vi "Linearity.vi"() -> ()   [LabVIEW 2014]
panel:
  out "mag of a.X1(w)+b.X2(w)":cluster{"-pi to pi":dbl[], "DTFT op":dbl[]}(graph)
  out "mag of DTFT{a.x1(n)+b.x2(n)}":cluster{"-pi to pi":dbl[], "DTFT op":dbl[]}(graph)
  out "a.X1(w)+b.X2(w)":cluster{"-pi to pi":dbl[], dbl[]}(graph)
  out "DTFT{a.x1(n)+b.x2(n)}":cluster{"-pi to pi":dbl[], "DTFT op":dbl[]}(graph)
  in  "Boolean":bool
  in  "b":dbl
  in  "x2(n)":dbl[](array[numeric])
  in  "a":dbl
  in  "x1(n)":dbl[](array[numeric])
  # "Instructions"
  # "1. Input the two sequences and the constants 'a' and 'b'\n2. verify the linearity property from the two graphs"
  # "if\nDTFT{x1(n)} ----> X1(w)\nDTFT{x2(n)} ----> X2(w)\nthen\nDTFT{a.x1(n)+b.x2(n)} ----> a.X1(w)+b.X2(w)"
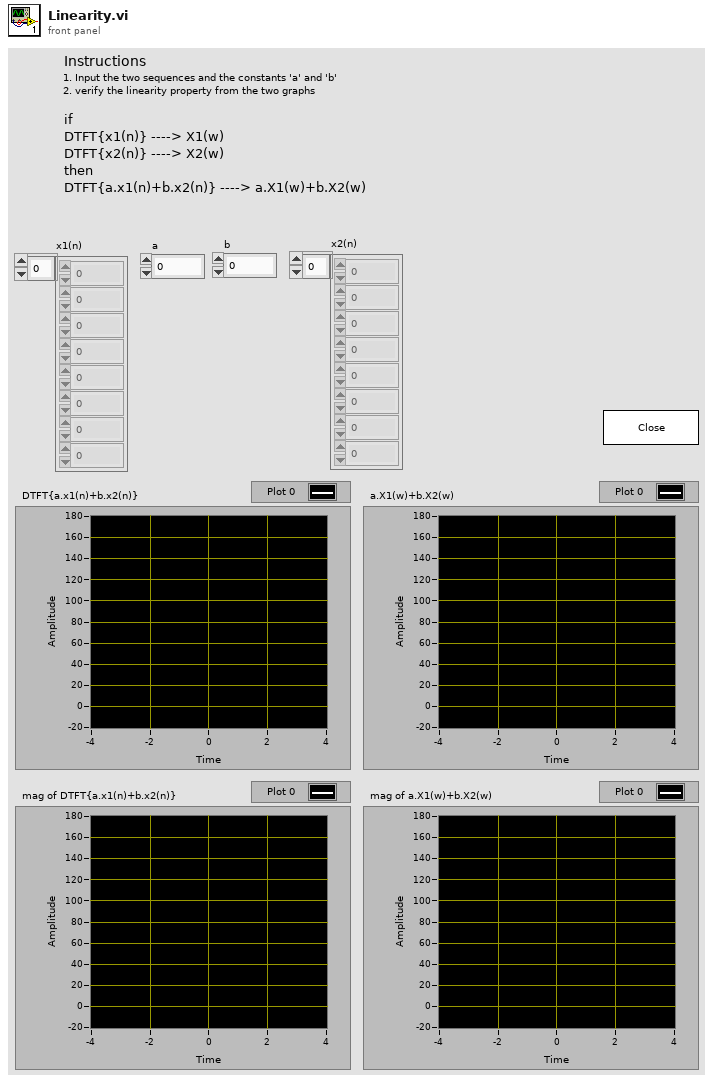
[diagram p1: front panel]
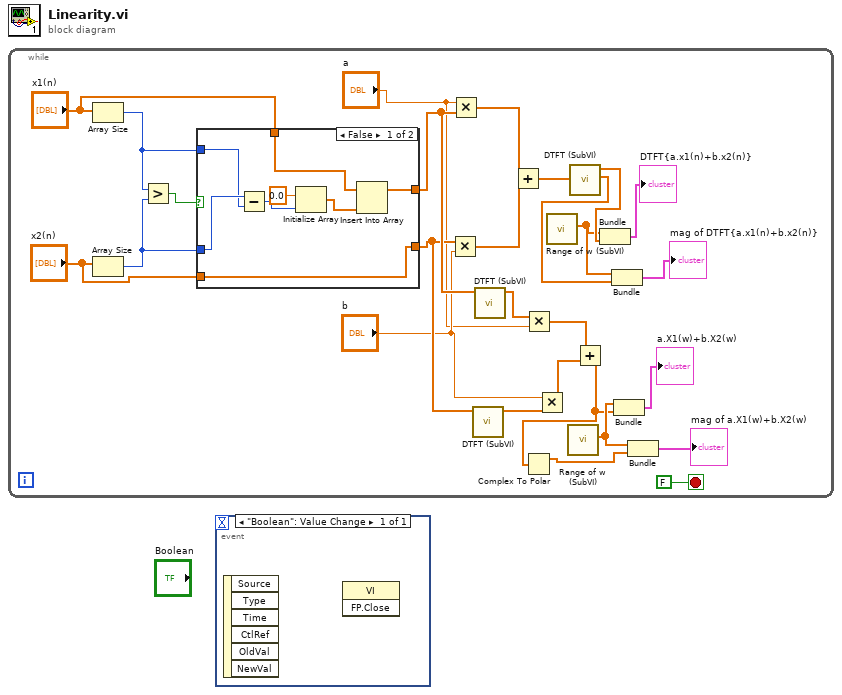
[diagram p0: block diagram]
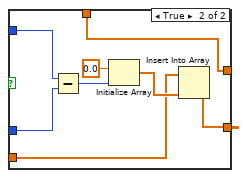
[diagram p2: hidden frame]
diagram:
  n1 = while {
    stop <- FALSE stop-if-true
    n2 = Array Size(array="x1(n)") -> (size(s)=w25:i32)
    n3 = Array Size(array="x2(n)") -> (size(s)=w24:i32)
    n4 = Greater?(x=w25, y=w24) -> (0:w26:bool)
    n5 = case shown="False" w26 {
      tunnel: w25 -> [w34 w43]
      tunnel: w24 -> [w35 w42]
      tunnel: "x2(n)" -> [w28 w38]
      tunnel: [w28 w37] -> w15
      tunnel: "x1(n)" -> [w30 w36]
      tunnel: [w29 w36] -> w16
      frame False {
        n6 = Subtract(x=w35, y=w34) -> (x-y=w33:i32)
        n7 = Initialize Array(0.0 ("element"), w33) -> (w31:dbl[])
        n8 = Insert Into Array(array=w30, new element=w31) -> (w29:dbl[])  [unwired: 1 in]
      }
      frame True {
        n9 = Subtract(x=w43, y=w42) -> (x-y=w41:i32)
        n10 = Initialize Array(0.0 ("element"), w41) -> (w39:dbl[])
        n11 = Insert Into Array(array=w38, new element=w39) -> (w37:dbl[])  [unwired: 1 in]
      }
    }
    n12 = Multiply(x=w15, y="b") -> (x*y=w18:dbl[])
    n13 = Multiply(x="a", y=w16) -> (x*y=w17:dbl[])
    n14 = call "DTFT (SubVI).vi"("ip array"=w15) -> ("DTFT op"=w11:cdb[])  [unwired: 9 in, 1 out]
    n15 = call "DTFT (SubVI).vi"("ip array"=w16) -> ("DTFT op"=w12:cdb[])  [unwired: 9 in, 1 out]
    n16 = Add(x=w17, y=w18) -> (x+y=w19:dbl[])
    n17 = Multiply(x=w12, y="a") -> (x*y=w20:cdb[])
    n18 = Multiply(x="b", y=w11) -> (x*y=w21:cdb[])
    n19 = call "Range of w (SubVI).vi"() -> ("-pi to pi"=w4:dbl[])  [unwired: 11 in]
    n20 = call "Range of w (SubVI).vi"() -> ("-pi to pi"=w5:dbl[])  [unwired: 11 in]
    n21 = call "DTFT (SubVI).vi"("ip array"=w19) -> ("Magnitude op"=w3:dbl[], "DTFT op"=w10:cdb[])  [unwired: 9 in]
    n22 = Add(x=w20, y=w21) -> (x+y=w1:cdb[])
    n23 = Complex To Polar(r * e^(i*theta)=w1) -> (r=w2:dbl[])  [unwired: 1 out]
    n24 = Bundle("-pi to pi"=w4, "DTFT op"=w10) -> (→"DTFT{a.x1(n)+b.x2(n)}":cluster{"-pi to pi":dbl[], "DTFT op":cdb[]})  [unwired: 1 in]
    n25 = Bundle("-pi to pi"=w4, "Magnitude op"=w3) -> (→"mag of DTFT{a.x1(n)+b.x2(n)}":cluster{"-pi to pi":dbl[], "Magnitude op":dbl[]})  [unwired: 1 in]
    n26 = Bundle("-pi to pi"=w5, w1) -> (→"a.X1(w)+b.X2(w)":cluster{"-pi to pi":dbl[], cdb[]})  [unwired: 1 in]
    n27 = Bundle("-pi to pi"=w5, w2) -> (→"mag of a.X1(w)+b.X2(w)":cluster{"-pi to pi":dbl[], dbl[]})  [unwired: 1 in]
  }
  n28 = event shown="[0] \"Boolean\": Value Change" {
    selector: _ -> [_]
    dyn-events: _ -> [_]
    timeout: _ -> [_]
    event "Boolean": Value Change {
      n29 = event-data() -> ()  [unwired: 1 in, 6 out]
      n30 = invoke class="VI" method="FP.Close"() -> ()  [unwired: 3 in, 3 out]
    }
  }
